vi "ScaleLink.vi"(7 "执行:调用时显示前面板":bool, 8 "曲线输入":dbl[][](array[numeric]), 9 "通量标尺":i32[](array[numeric]), 10 "通量名称":string[](array[string]), 11 "通量输入":dbl[](array[numeric])) -> (3 "通量输出":dbl[](array[numeric]))   [LabVIEW 2020]
uses:
  <vilib>/Analysis/polynomials.llb/Scalar Polynomial Evaluation (DBL).vi
  <vilib>/Analysis/NI_AALPro.lvlib
panel:
  out "ScaleLink曲线":dbl[][](graph)
  in  "待接量程":u16(ring) items=["电流1a", "电流2a"]
  in  "子量程":u16(ring) items=["电流1a", "电流2a"]
  out "待接量程":dbl
  out "子量程":dbl
  in  "开始衔接":bool
  out "衔接系数":dbl[](array[numeric]) min=0.0 max=127.0 format="%#.2f"
  out "最新衔接点：":dbl
  out "前面板窗口:打开":bool
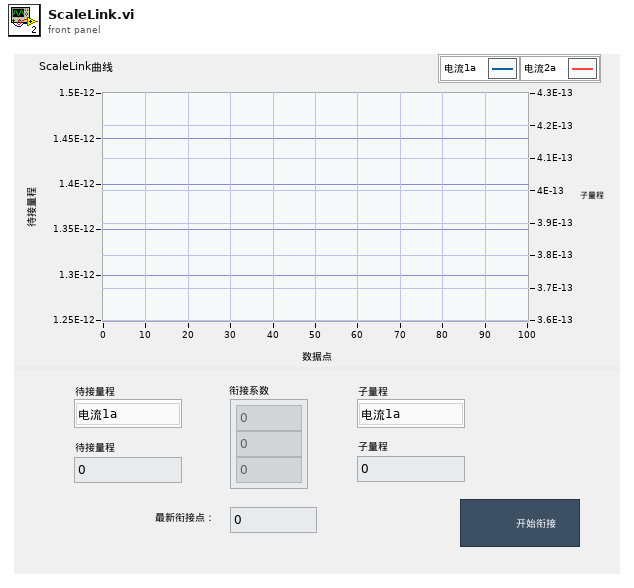
[diagram p1: front panel]
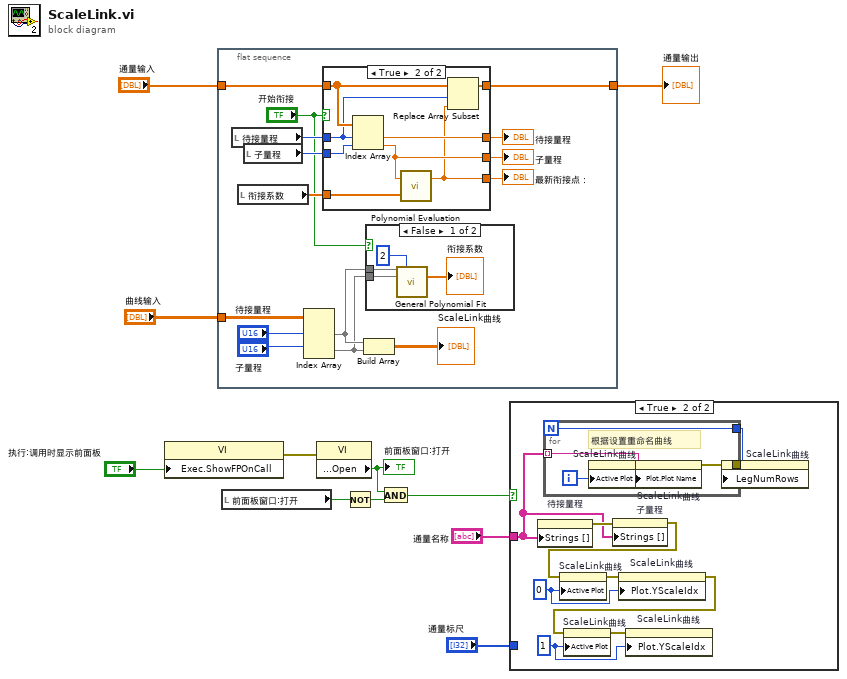
[diagram p0: block diagram]
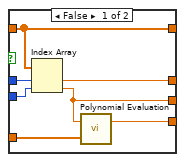
[diagram p4: hidden frame]
diagram:
  n1 = property class="VI"("Exec.ShowFPOnCall"="执行:调用时显示前面板") -> (error out=w10:errorcluster)  [unwired: 2 in, 1 out]
  n2 = flat-sequence {
    tunnel: "通量输入" -> [w26]
    tunnel: [w24] -> w1
    tunnel: "曲线输入" -> [w25]
    frame #0 {
      n3 = local read "待接量程"() -> (w21:u16)
      n4 = local read "衔接系数"() -> (w17:dbl[])
      n5 = local read "子量程"() -> (w20:u16)
      n6 = Index Array(array=w25, index (row) #1="待接量程", index (row) #2="子量程") -> (element #1=w16:dbl[], element #2=w15:dbl[])  [unwired: 2 in]
      n7 = case shown="True" "开始衔接" {
        tunnel: w26 -> [w35 w45]
        tunnel: [w35 w42] -> w24
        tunnel: w21 -> [w37 w44]
        tunnel: w20 -> [w36 w43]
        tunnel: [w34 w41] -> w19
        tunnel: [w32 w39] -> w18
        tunnel: w17 -> [w33 w40]
        tunnel: [w31 w38] -> w13
        frame False {
          n8 = Index Array(array=w35, index #1=w37, index #2=w36) -> (element #1=w34:dbl, element #2=w32:dbl)
          n9 = call-poly <vilib>:"Polynomial Evaluation.vi"("P(x)"=w33, "a"=w32) -> ("P(a)"=w31:dbl)  [unwired: 1 out]
        }
        frame True {
          n10 = Index Array(array=w45, index #1=w44, index #2=w43) -> (element #1=w41:dbl, element #2=w39:dbl)
          n11 = call-poly <vilib>:"Polynomial Evaluation.vi"("P(x)"=w40, "a"=w39) -> ("P(a)"=w38:dbl)  [unwired: 1 out]
          n12 = Replace Array Subset(array=w45, new element=w38, index=w44) -> (w42:dbl[])
        }
      }
      "待接量程" <- w19
      "子量程" <- w18
      "最新衔接点：" <- w13
      n13 = Build Array(w16, w15) -> (→"ScaleLink曲线":dbl[][])
      n14 = case shown="False" "开始衔接" {
        tunnel: w16 -> [w30 _]
        tunnel: w15 -> [w29 _]
        frame False {
          n15 = call <vilib>:"General Polynomial Fit.vi"("Y"=w30, "polynomial order"=2, "X"=w29) -> ("Polynomial Coefficients"=→"衔接系数":dbl[])  [unwired: 9 in, 3 out]
        }
        frame True {
        }
      }
    }
  }
  n16 = local read "前面板窗口:打开"() -> (w8:bool)
  n17 = property class="VI"(error in=w10) -> ("Front Panel.Open"=w6:bool)  [unwired: 1 in, 2 out]
  "前面板窗口:打开" <- w6
  n18 = Not(x=w8) -> (.not. x?=w7:bool)
  n19 = And(x=w6, y=w7) -> (x .and. y?=w5:bool)
  n20 = case shown="True" w5 {
    tunnel: "通量名称" -> [_ w46]
    tunnel: "通量标尺" -> [_ _]
    frame False {
    }
    frame True {
      w53 = u32 1 ("活动曲线")
      w54 = u32 0 ("活动曲线")
      n21 = property on="待接量程" class="Ring (strict)"("Strings []"=w46) -> (error out=w50:errorcluster)  [unwired: 2 in, 1 out]
      n22 = for {
        N -> [w57]
        tunnel: w46 -> [w58] mode=indexing
        tunnel: [w57] -> w49
        tunnel: [w56] -> w48
        i -> [w60]
        # "根据设置重命名曲线"
        n23 = property on="ScaleLink曲线" class="WFGraph (strict)"("Active Plot"=w60) -> (error out=w59:errorcluster)  [unwired: 2 in, 1 out]
        n24 = property on="ScaleLink曲线" class="WFGraph (strict)"(error in=w59, "Plot.Plot Name"=w58) -> (error out=w56:errorcluster)  [unwired: 1 in, 1 out]
      }
      n25 = property on="子量程" class="Ring (strict)"(error in=w50, "Strings []"=w46) -> (error out=w55:errorcluster)  [unwired: 1 in, 1 out]
      n26 = property on="ScaleLink曲线" class="WFGraph (strict)"(error in=w55, "Active Plot"=w54) -> (error out=w47:errorcluster)  [unwired: 1 in, 1 out]
      n27 = property on="ScaleLink曲线" class="WFGraph (strict)"(error in=w47, "Plot.YScaleIdx"=w54) -> (error out=w52:errorcluster)  [unwired: 1 in, 1 out]
      n28 = property on="ScaleLink曲线" class="WFGraph (strict)"(error in=w52, "Active Plot"=w53) -> (error out=w51:errorcluster)  [unwired: 1 in, 1 out]
      n29 = property on="ScaleLink曲线" class="WFGraph (strict)"(error in=w51, "Plot.YScaleIdx"=w53) -> ()  [unwired: 1 in, 2 out]
      n30 = property on="ScaleLink曲线" class="WFGraph (strict)"(error in=w48, "LegNumRows"=w49) -> ()  [unwired: 1 in, 2 out]
    }
  }
  "通量输出" <- w1
